vi "Set Steer Angles (Relative).vi"(8 "Rear Right":dbl, 9 "Rear Left":dbl, 10 "Front Right":dbl, 11 "Front Left":dbl) -> ()   [LabVIEW 2011]
uses:
  Globals/Jaguar Commands.vi
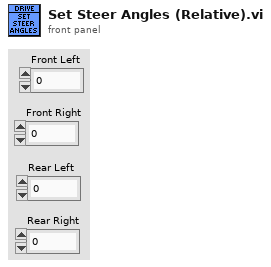
[diagram p1: front panel]
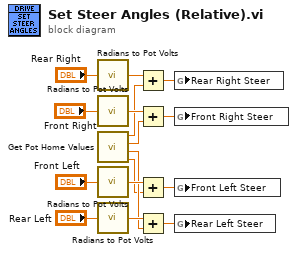
[diagram p0: block diagram]
diagram:
  n1 = call "Radians to Pot Volts.vi"("Angle In"="Rear Right") -> ("Pot Delta Out"=w13:dbl)
  n2 = call "Radians to Pot Volts.vi"("Angle In"="Front Right") -> ("Pot Delta Out"=w15:dbl)
  n3 = call "Get Pot Home Values.vi"() -> ("Front Left"=w5:dbl, "Rear Left"=w6:dbl, "Front Right"=w7:dbl, "Rear Right"=w8:dbl)  [unwired: 8 in]
  n4 = call "Radians to Pot Volts.vi"("Angle In"="Front Left") -> ("Pot Delta Out"=w16:dbl)
  n5 = call "Radians to Pot Volts.vi"("Angle In"="Rear Left") -> ("Pot Delta Out"=w14:dbl)
  n6 = Add(x=w13, y=w8) -> (x+y=w1:dbl)
  n7 = Add(x=w15, y=w7) -> (x+y=w3:dbl)
  n8 = Add(x=w16, y=w5) -> (x+y=w4:dbl)
  n9 = Add(x=w14, y=w6) -> (x+y=w2:dbl)
  n10 = global write "Jaguar Commands.vi" "Rear Right Steer"(w1) -> ()
  n11 = global write "Jaguar Commands.vi" "Front Right Steer"(w3) -> ()
  n12 = global write "Jaguar Commands.vi" "Front Left Steer"(w4) -> ()
  n13 = global write "Jaguar Commands.vi" "Rear Left Steer"(w2) -> ()
